vi "Read Data.vi"(8 "error in (no error)":errorcluster, 10 "Name":string, 11 "Observable Actor in":refnum<class "Observable Actor.lvclass">) -> (0 "error out":errorcluster, 1 "found":bool, 2 "Data":refnum<class "AbstractData.lvclass">, 3 "Observable Actor out":refnum<class "Observable Actor.lvclass">)   [LabVIEW 2014, in "Observable Actor.lvlib" / "Observable Actor.lvclass"]
uses:
  Observable Actor.lvclass
  Model/Data/AbstractData/AbstractData.lvclass
  Observable Actor.lvclass/Observable Actor.ctl
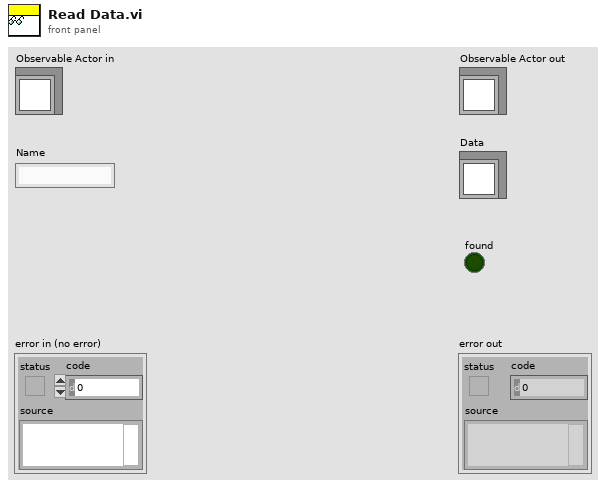
[diagram p1: front panel]
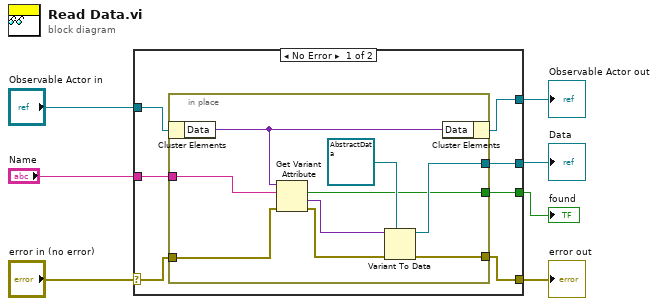
[diagram p0: block diagram]
diagram:
  n1 = case shown="No Error" "error in (no error)" {
    selector: "error in (no error)" -> [w10 w24]
    tunnel: [w9 w24] -> w6
    tunnel: [w12 w25] -> w3
    tunnel: "Observable Actor in" -> [w13 w25]
    tunnel: [w11 _] -> w4
    tunnel: "Name" -> [w14 _]
    tunnel: [w8 _] -> w1
    frame No Error {
      n2 = in-place {
        in-place-border: w14 -> [w21]
        in-place-border: [w20] -> w11
        in-place-border: [w18] -> w9
        in-place-border: w10 -> [w17]
        in-place-border: [w15] -> w8
        n3 = in-place-cluster #1(w13) -> ("Data"=w22:variant)
        n4 = Get Variant Attribute(Variant=w22, name=w21, error in=w17) -> (found=w15:bool, value=w23:variant, error out=w19:errorcluster)  [unwired: 1 in, 1 out]
        n5 = Variant To Data(error in=w19, type=refnum<class "AbstractData.lvclass"> refnum ("AbstractData.lvclass"), Variant=w23) -> (data=w20:refnum<class "AbstractData.lvclass">, error out=w18:errorcluster)
        n6 = in-place-cluster #1("Data"=w22) -> (w12:refnum<class "Observable Actor.lvclass">)
      }
    }
    frame Error {
    }
  }
  "error out" <- w6
  "Data" <- w4
  "Observable Actor out" <- w3
  "found" <- w1
